vi "Hasscan_advanced_output_bus_line_raw.vi"(8 "error in (no error)":errorcluster, 11 "OneOfTemplate in":refnum<class "niswitch_grpc_RouteScanAdvancedOutputRequest_scan_advanced_output_bus_line_enum.lvclass">) -> (0 "error out":errorcluster, 2 "Has Data?":bool, 3 "OneOfTemplate out":refnum<class "niswitch_grpc_RouteScanAdvancedOutputRequest_scan_advanced_output_bus_line_enum.lvclass">)   [LabVIEW 2021, in "NI Switch_client.lvlib" / "niswitch_grpc_RouteScanAdvancedOutputRequest_scan_advanced_output_bus_line_enum.lvclass"]
uses:
  niswitch_grpc_RouteScanAdvancedOutputRequest_scan_advanced_output_bus_line_enum.lvclass
  niswitch_grpc_RouteScanAdvancedOutputRequest_scan_advanced_output_bus_line_enum.lvclass/niswitch_grpc_RouteScanAdvancedOutputRequest_scan_advanced_output_bus_line_enum.ctl
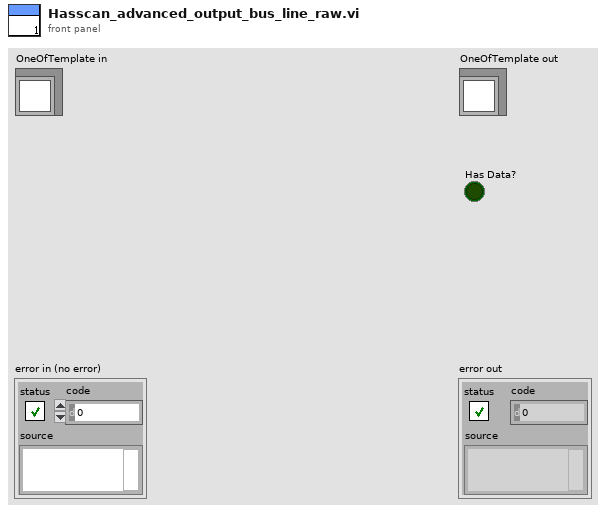
[diagram p1: front panel]
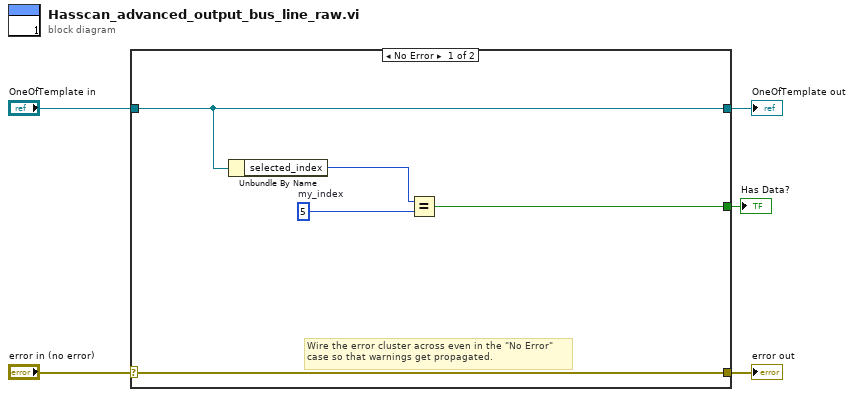
[diagram p0: block diagram]
diagram:
  n1 = case shown="No Error" "error in (no error)" {
    selector: "error in (no error)" -> [w10 w12]
    tunnel: [w10 w12] -> w4
    tunnel: [w9 w11] -> w2
    tunnel: "OneOfTemplate in" -> [w9 w11]
    tunnel: [w6 _] -> w1
    frame No Error {
      w7 = 5  # my_index
      # "Wire the error cluster across even in the \"No Error\"\ncase so that warnings get propagated."
      n2 = Unbundle By Name(w9) -> ("selected_index"=w8:i32)
      n3 = Equal?(x=w8, y=w7) -> (x = y?=w6:bool)
    }
    frame Error {
    }
  }
  "error out" <- w4
  "OneOfTemplate out" <- w2
  "Has Data?" <- w1
